vi "Recursive Add Item References to Map.vi"(8 "error in (no error)":errorcluster, 10 "ProjectItem Refnum":refnum<vi>, 11 "Icon Decorator in":refnum<class "Icon Decorator.lvclass">) -> (0 "error out":errorcluster, 3 "Icon Decorator out":refnum<class "Icon Decorator.lvclass">)   [LabVIEW 2020, in "Icon Decorator.lvclass"]
uses:
  Icon Decorator.lvclass
  Icon Decorator.lvclass/Icon Decorator.ctl
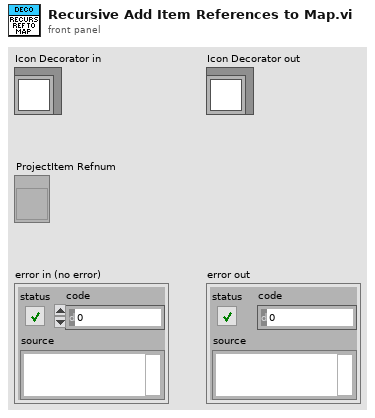
[diagram p1: front panel]
types:
  T1 = typedef "ItemRef.ctl" = u64
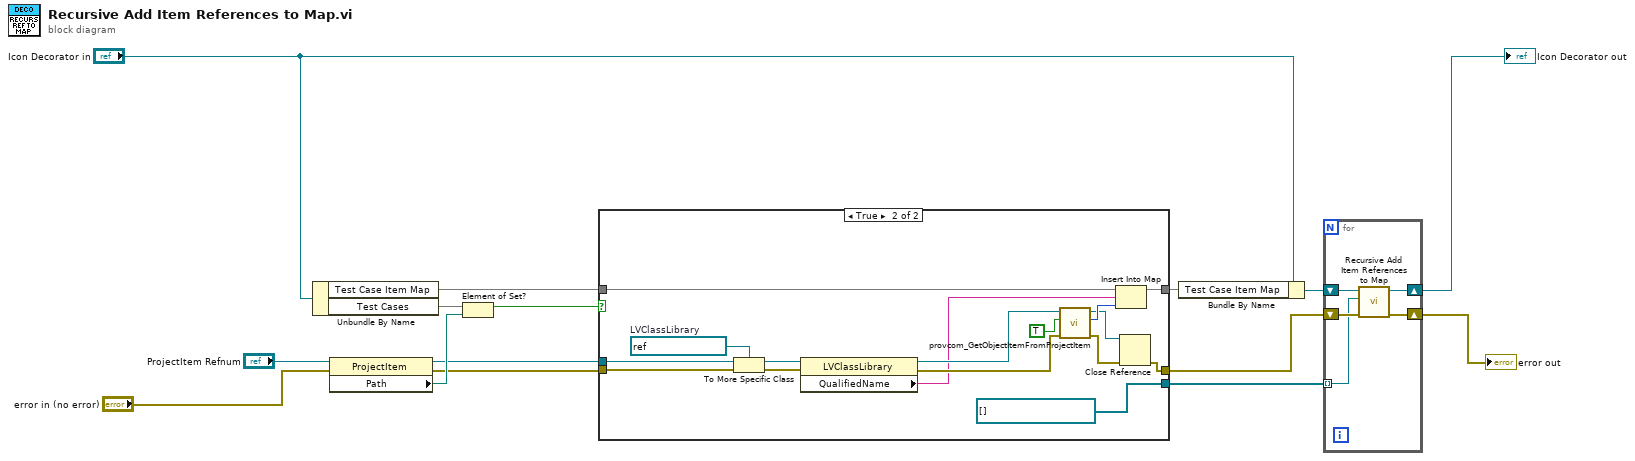
[diagram p0: block diagram]
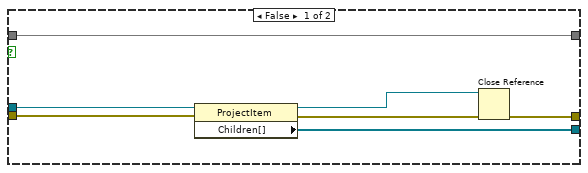
[diagram p2: hidden frame]
diagram:
  n1 = Unbundle By Name("Icon Decorator in") -> ("Test Case Item Map"=w10:map{string, T1}, "Test Cases"=w9:set{path})
  n2 = property class="ProjectItem"(reference="ProjectItem Refnum", error in="error in (no error)") -> (reference out=w3:refnum<vi>, error out=w2:errorcluster, "Path"=w4:path)
  n3 = Element of Set?(10:w4, 11:w9) -> (3:w12:bool)
  n4 = case shown="True" w12 {
    tunnel: w10 -> [w21 w37]
    tunnel: w3 -> [w18 w36]
    tunnel: w2 -> [w17 w29]
    tunnel: [w22 w32] -> w8
    tunnel: [w21 w31] -> w13
    tunnel: [w16 refnum<vi>[] [] ("Children[]")] -> w1
    frame False {
      n5 = property class="ProjectItem"(reference=w18, error in=w17) -> (reference out=w20:refnum<vi>, error out=w19:errorcluster, "Children[]"=w16:refnum<vi>[])
      n6 = Close Reference(reference=w20, error in (no error)=w19) -> (error out=w22:errorcluster)
    }
    frame True {
      w28 = refnum<vi> refnum  # LVClassLibrary
      n7 = To More Specific Class(target class=w28, reference=w36, error in=w29) -> (specific class reference=w30:refnum<vi>, error out=w26:errorcluster)
      n8 = property class="LVClassLibrary"(reference=w30, error in=w26) -> (reference out=w27:refnum<vi>, error out=w25:errorcluster, "QualifiedName"=w24:string)
      n9 = call <resource>:"provcom_GetObjectItemFromProjectItem.vi"("error in (no error)"=w25, "bind? (Y)"=TRUE, "ProjectItem"=w27) -> ("error out"=w33:errorcluster, "ObjectItem"=w35:T1, "dup ProjectItem"=w34:refnum<vi>)  [unwired: 6 in]
      n10 = Insert Into Map(map in=w37, key=w24, value=w35) -> (map out=w31:map{string, T1})  [unwired: 2 out]
      n11 = Close Reference(reference=w34, error in (no error)=w33) -> (error out=w32:errorcluster)
    }
  }
  n12 = Bundle By Name(cluster="Icon Decorator in", "Test Case Item Map"=w13) -> (w6:refnum<class "Icon Decorator.lvclass">)
  n13 = for {
    shift-right: [w42] -> w7
    shift-left: w8 -> [w43]
    shift-right: [w40] -> w5
    shift-left: w6 -> [w41]
    tunnel: w1 -> [w39] mode=indexing
    n14 = call "Recursive Add Item References to Map.vi"("error in (no error)"=w43, "ProjectItem Refnum"=w39, "Icon Decorator in"=w41) -> ("error out"=w42:errorcluster, "Icon Decorator out"=w40:refnum<class "Icon Decorator.lvclass">)  [unwired: 7 in]
  }
  "Icon Decorator out" <- w5
  "error out" <- w7
